vi "calculate stack duration.vi"(8 "error in (no error)":errorcluster, 11 "Autofocus in":refnum<class "Autofocus.lvclass">) -> (0 "error out":errorcluster, 3 "Autofocus out":refnum<class "Autofocus.lvclass">)   [LabVIEW 2012, in "Autofocus.lvclass"]
uses:
  Autofocus.lvclass
  Autofocus.lvclass/Autofocus.ctl
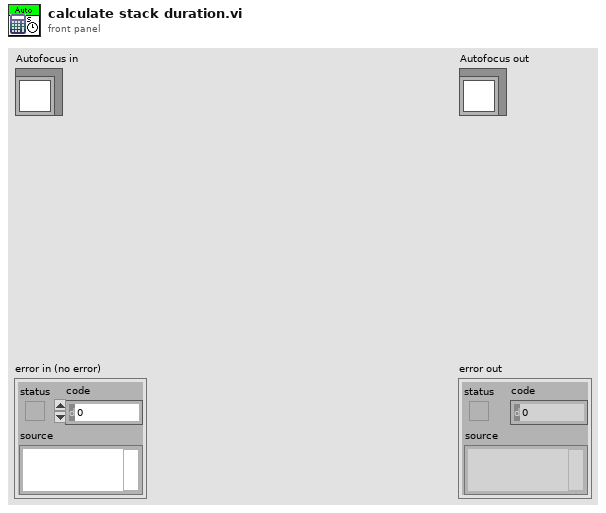
[diagram p1: front panel]
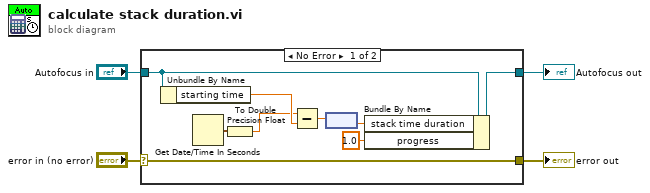
[diagram p0: block diagram]
diagram:
  n1 = case shown="No Error" "error in (no error)" {
    selector: "error in (no error)" -> [w13 w15]
    tunnel: [w13 w15] -> w3
    tunnel: [w7 w14] -> w1
    tunnel: "Autofocus in" -> [w8 w14]
    frame No Error {
      n2 = Unbundle By Name(w8) -> ("starting time"=w6:dbl)
      n3 = Get Date/Time In Seconds() -> (seconds since 1Jan1904=w9:timestamp)
      n4 = To Double Precision Float(number=w9) -> (double precision float=w5:dbl)
      n5 = Subtract(x=w5, y=w6) -> (x-y=w11:dbl)
      n6 = node(w11) -> (w12:dbl[unit])
      n7 = Bundle By Name(cluster=w8, "stack time duration"=w12, "progress"=1.0 ("Runtime cluster.Stack.progress")) -> (w7:refnum<class "Autofocus.lvclass">)
    }
    frame Error {
    }
  }
  "error out" <- w3
  "Autofocus out" <- w1
